vi "List Manager (main).vi"() -> (1 "Open Device":bool, 3 "COM port":string)   [LabVIEW 2010]
panel:
  in  "first run":bool
  in  "refresh flag":bool
  in  "cancel":bool
  in  "refresh":bool
  out "devices and versions list":T1(array[cluster])
  in  "Refresh 2":bool
  in  "Table":i32(listbox)=-1 caption="Harp devices list:"
  in  "Double click an Harp device to:":T2(radio)
  # "Available Harp Devices"
  # "Double click an Harp device line to update User Device Name."
  # "Harp is a family of hardware synchronized devices integrating wireless 9-axis motion sensors,\nLoad Cells readers, RGB controllers, Behavior boards, TTL Synchronizers, PWM generator, etc.\nIf want to know more about any of the devices, contact hardware@neuro.fchampalimaud.org"
  # "Device Name Given By the User"
  # "Double click an Harp device to:"
  # "Double click an Harp device to:"
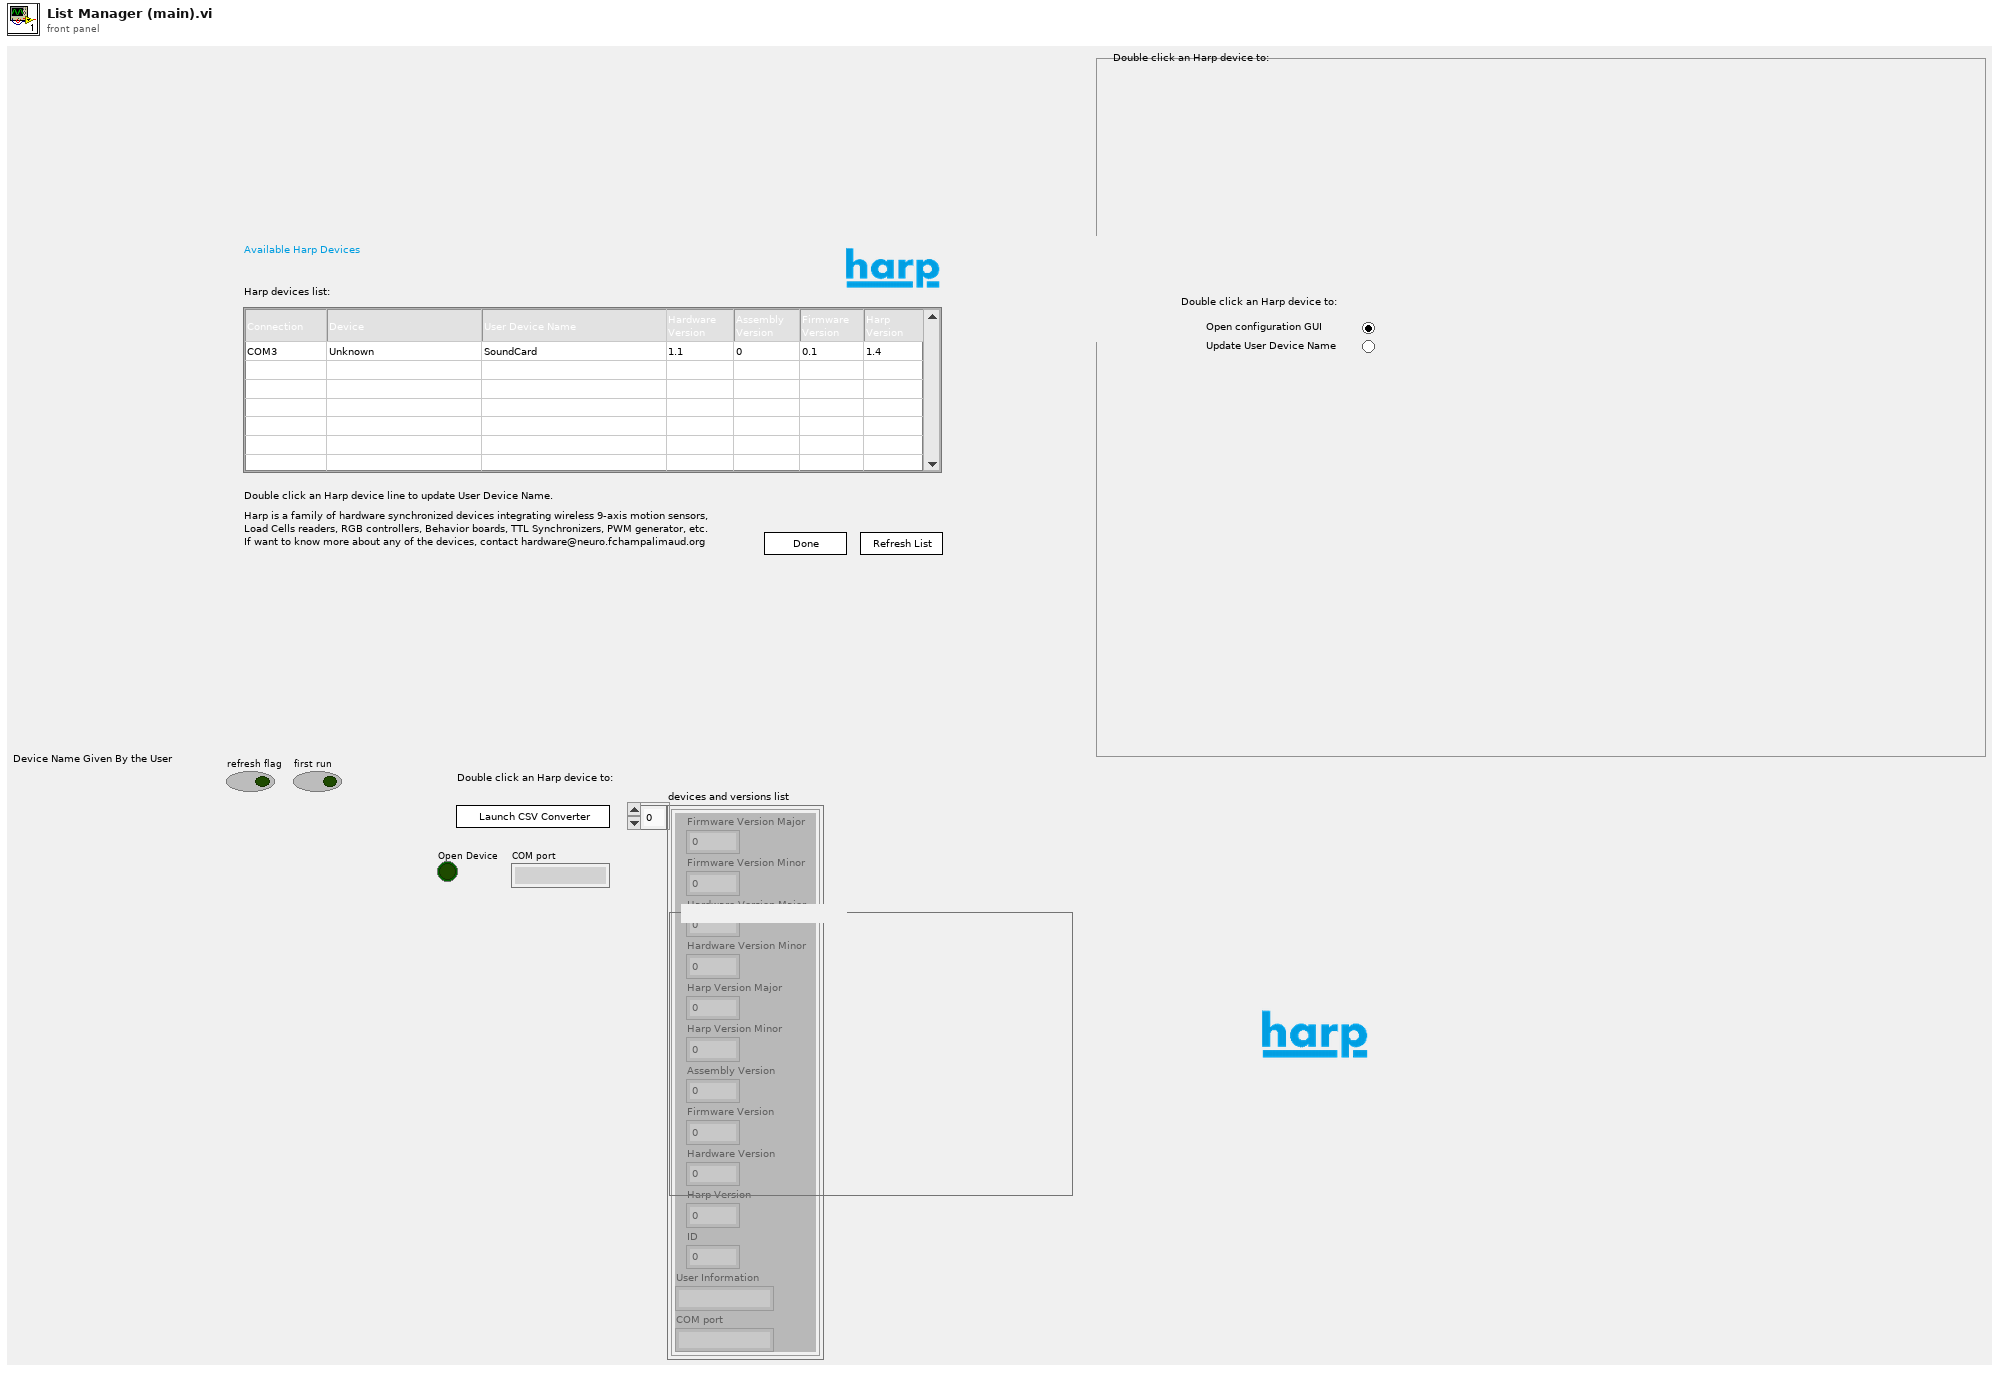
[diagram p1: front panel]
types:
  T1 = cluster{"Firmware Version Major":u8, "Firmware Version Minor":u8, "Hardware Version Major":u8, "Hardware Version Minor":u8, "Harp Version Major":u8, "Harp Version Minor":u8, "Assembly Version":u8, "Firmware Version":dbl, "Hardware Version":dbl, "Harp Version":dbl, "ID":u16, "User Information":string, "COM port":string}[]
  T2 = enum32{"Open configuration GUI", "Update User Device Name"}
  T3 = cluster{"Firmware Version Major":u8, "Firmware Version Minor":u8, "Hardware Version Major":u8, "Hardware Version Minor":u8, "Harp Version Major":u8, "Harp Version Minor":u8, "Assembly Version":u8, "Firmware Version":dbl, "Hardware Version":dbl, "Harp Version":dbl, "ID":u16, "User Information":string, "COM port":string}
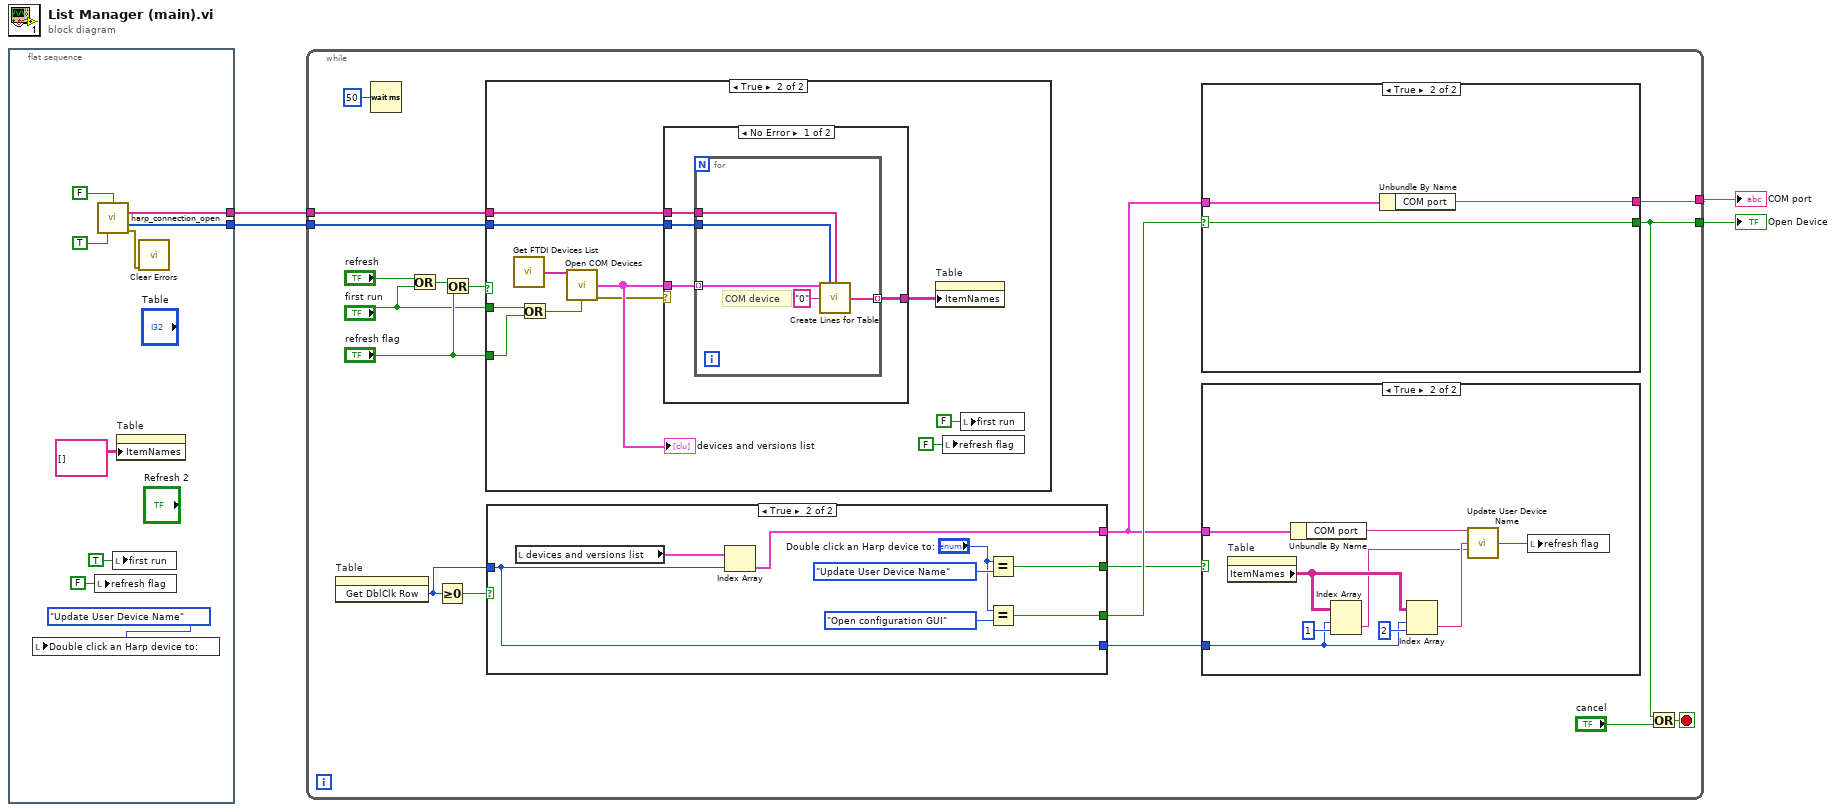
[diagram p0: block diagram]
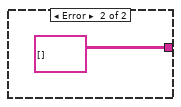
[diagram p6: hidden frame]
diagram:
  n1 = flat-sequence {
    tunnel: [w11] -> w4
    tunnel: [w10] -> w3
    frame #0 {
      n2 = local write "Double click an Harp device to:"(T2."Update User Device Name" ("y")) -> ()
      n3 = local write "refresh flag"(FALSE ("refresh flag")) -> ()
      n4 = call "harp_connection_open.vi"("launch dialog"=FALSE, "get lists only"=TRUE) -> ("Devices Name List"=w11:string[], "Devices WhoAmI List"=w10:u16[], "error out"=w9:errorcluster)  [unwired: 8 in, 3 out]
      n5 = local write "first run"(TRUE ("first run")) -> ()
      n6 = property on="Table" class="MCListbox (strict)"("ItemNames"=string[][] [] ("Item Names")) -> ()  [unwired: 2 in, 2 out]
      n7 = call <vilib>:"Clear Errors.vi"("error in (no error)"=w9) -> ()  [unwired: 6 in, 1 out]
    }
  }
  n8 = while {
    tunnel: w4 -> [w31]
    tunnel: w3 -> [w30]
    tunnel: [w16] -> w2
    tunnel: [w24] -> w1
    stop <- w17 stop-if-true
    n9 = invoke on="Table" class="MCListbox (strict)" method="Get DblClk Row"() -> ("Get Double-clicked Row"=w27:i32)  [unwired: 3 in, 2 out]
    n10 = Wait (ms)(milliseconds to wait=u32 50) -> ()  [unwired: 1 out]
    n11 = Or(x="refresh", y="first run") -> (x .or. y?=w29:bool)
    n12 = Greater Or Equal To 0?(x=w27) -> (x >= 0?=w26:bool)
    n13 = Or(x=w29, y="refresh flag") -> (x .or. y?=w18:bool)
    n14 = case shown="True" w18 {
      tunnel: w31 -> [_ w60]
      tunnel: w30 -> [_ w59]
      tunnel: "first run" -> [_ w57]
      tunnel: "refresh flag" -> [_ w55]
      frame False {
      }
      frame True {
        n15 = call "Get FTDI Devices List.vi"() -> ("FTDI Serial Ports"=w64:string[])  [unwired: 13 in, 2 out]
        n16 = Or(x=w57, y=w55) -> (x .or. y?=w56:bool)
        n17 = call "Open COM Devices.vi"("com ports list"=w64, "Wait 3s?"=w56) -> ("devices and versions list"=w63:T1, "error out"=w62:errorcluster)  [unwired: 12 in]
        "devices and versions list" <- w63
        n18 = case shown="No Error" w62 {
          tunnel: w63 -> [w68 _]
          tunnel: [w67 string[][] [] ("line")] -> w61
          tunnel: w60 -> [w66 _]
          tunnel: w59 -> [w65 _]
          frame No Error {
            n19 = for {
              tunnel: w68 -> [w73] mode=indexing
              tunnel: [w71] -> w67 mode=indexing
              tunnel: w66 -> [w70]
              tunnel: w65 -> [w69]
              # "COM device"
              n20 = call "Create Lines for Table.vi"("versions"=w73, "Devices WhoAmI List"=w69, "Devices Name List"=w70, "connection type"="0") -> ("line"=w71:string[])  [unwired: 11 in]
            }
          }
          frame Error {
          }
        }
        n21 = property on="Table" class="MCListbox (strict)"("ItemNames"=w61) -> ()  [unwired: 2 in, 2 out]
        n22 = local write "refresh flag"(FALSE ("refresh flag")) -> ()
        n23 = local write "first run"(FALSE ("first run")) -> ()
      }
    }
    n24 = case shown="True" w26 {
      selector: w26 -> [w45 _]
      tunnel: w27 -> [_ w46]
      tunnel: [w45 w49] -> w23
      tunnel: [w45 w48] -> w25
      tunnel: [_ w46] -> w19
      tunnel: [_ w47] -> w22
      frame False {
      }
      frame True {
        n25 = local read "devices and versions list"() -> (w53:T1)
        n26 = Index Array(array=w53, index=w46) -> (element=w47:T3)
        n27 = Equal?(x="Double click an Harp device to:", y=T2."Update User Device Name") -> (x = y?=w49:bool)
        n28 = Equal?(x="Double click an Harp device to:", y=T2."Open configuration GUI") -> (x = y?=w48:bool)
      }
    }
    n29 = case shown="True" w25 {
      selector: w25 -> [w41 w43]
      tunnel: w22 -> [_ w44]
      tunnel: [w41 w43] -> w16
      tunnel: [_ w42] -> w24
      frame False {
      }
      frame True {
        n30 = Unbundle By Name(w44) -> ("COM port"=w42:string)
      }
    }
    n31 = case shown="True" w23 {
      tunnel: w22 -> [_ w40]
      tunnel: w19 -> [_ w36]
      frame False {
      }
      frame True {
        n32 = property on="Table" class="MCListbox (strict)"() -> ("ItemNames"=w35:string[][])  [unwired: 2 in, 2 out]
        n33 = Unbundle By Name(w40) -> ("COM port"=w39:string)
        n34 = Index Array(array=w35, index (row)=w36, index (col)=1 ("disabled index (col)")) -> (element=w33:string)
        n35 = Index Array(array=w35, index (row)=w36, index (col)=2 ("disabled index (col)")) -> (element=w34:string)
        n36 = call "Update User Device Name.vi"("Serial Port"=w39, "Current:"=w34, "Device:"=w33) -> ("Update Done"=w32:bool)  [unwired: 12 in]
        n37 = local write "refresh flag"(w32) -> ()
      }
    }
    n38 = Or(x=w16, y="cancel") -> (x .or. y?=w17:bool)
  }
  "Open Device" <- w2
  "COM port" <- w1
